vi "calc filter scale.vi"() -> ()   [LabVIEW 2015]
uses:
  <vilib>/Analysis/NI_AALBase.lvlib
panel:
  out "Waveform Graph 2":i32[](graph)
  out "Waveform Graph":i32[](graph)
  out "x*y 2":i32 format="%.0f (x%x)"
  out "x*y":dbl format="%#_10g"
  in  "Input":i32 format="%d (b%b) (x%x)"
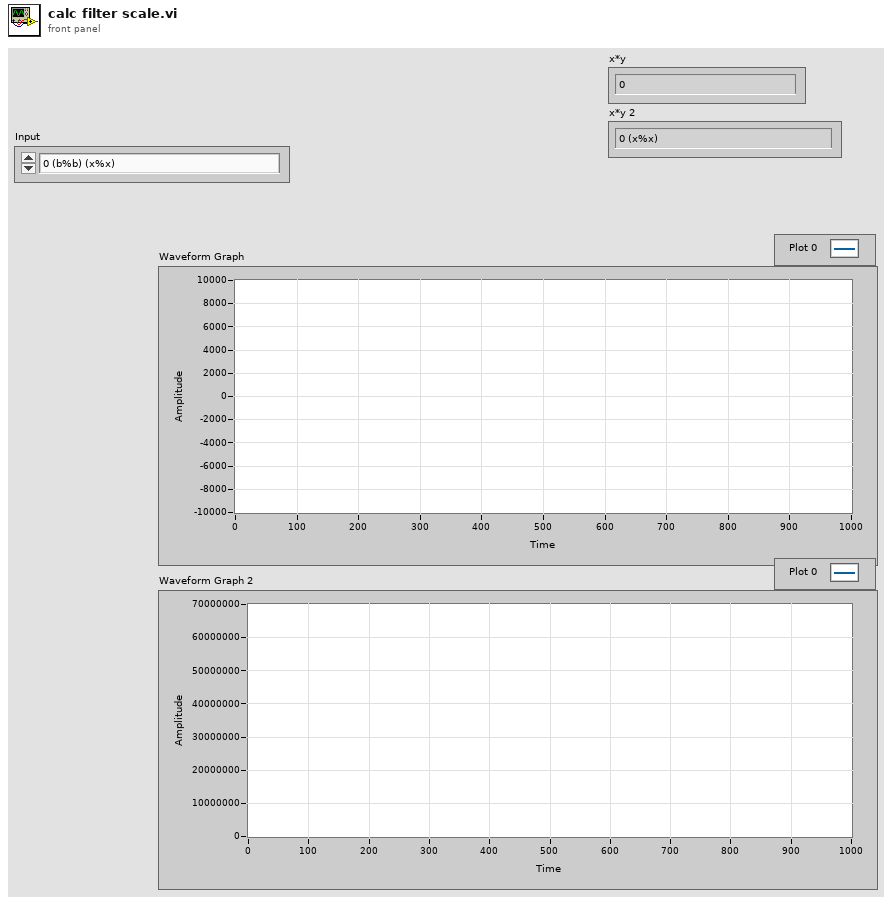
[diagram p1: front panel]
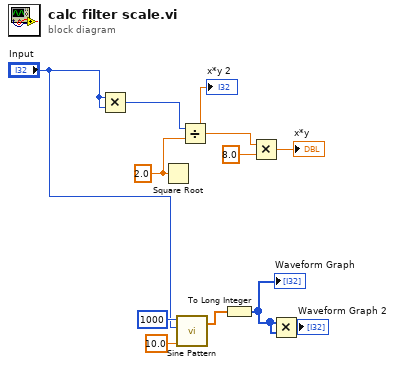
[diagram p0: block diagram]
diagram:
  w8 = 2.0 ("x")
  n1 = Multiply(x="Input", y="Input") -> (x*y=w9:i32)
  n2 = Square Root(x=w8) -> ()  [unwired: 1 out]
  n3 = call <vilib>:"Sine Pattern.vi"("cycles"=10.0, "amplitude"="Input", "samples"=1000) -> ("Sinusoidal Pattern"=w3:dbl[])  [unwired: 1 in, 1 out]
  n4 = Divide(x=w9, y=w8) -> (x/y=w7:dbl)
  "x*y 2" <- w7
  n5 = To Long Integer(number=w3) -> (32bit integer=w2:i32[])
  "Waveform Graph" <- w2
  n6 = Multiply(x=w7, y=8.0) -> (x*y=→"x*y":dbl)
  n7 = Multiply(x=w2, y=w2) -> (x*y=→"Waveform Graph 2":i32[])
